vi "LoadFromLVSET.vi"(8 "Error In":errorcluster, 10 "No of Active\nModules":i32=1, 11 "File Path":path) -> (0 "Error Out":errorcluster, 3 "System Paramters For Each Module":T1[](array[typedef]) {"sync_freq_div" items=["1"=1, "2"=2, "4"=4]; "cfd_zc_level" min=-96 max=96 step=0.1 format="%#_3g"; "cfd_limit_low" min=-500 max=0 step=0.1 format="%#_3g"; "sync_zc_level" min=-96 max=96 step=0.1 format="%#_3g"; "sync_threshold" min=-500 max=-20 step=0.1 format="%#_3g"; "tac_limit_low" format="%.3g"; "tac_limit_high" min=0 max=100 step=0.1 format="%.3g"; "collect_time" min=1e-07 max=100000 step=0.001; "tac_offset" min=0 max=100 step=0.1 format="%.4g"; "tac_gain" min=1 max=15 step=1; "tac_range" format="%^#_6g"})   [LabVIEW 2017]
doc: "This convenience VI loads the user setting parameter such as TAC range, Sync Threshold and CFD Limit Low from a given LVSET file.\nIs no file specified the default file will be used, located at: \"C:\\BHdata\\SPCM\\SPCDefaultVal.lvset\"\n\ninfo@becker-hickl.com"
uses:
  Example_Controls/UserInput.ctl
panel:
  # "TAC / Time Range"
  # "CFD"
  # "(start)"
  # "SYNC"
  # "(stop)"
  # "range"
  # "gain"
  # "threshold(LL)"
  # "offset"
  # "limit high"
  # "limit low"
  # "zero cross(ZC)"
  # "Collection Time"
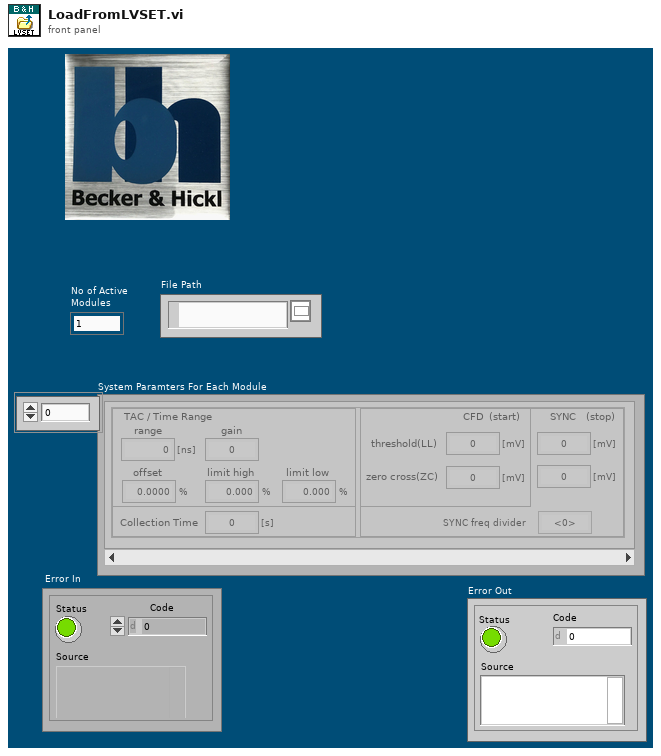
[diagram p1: front panel]
types:
  T1 = typedef "UserInput.ctl" = cluster{"tac_range":sgl, "tac_gain":i16, "tac_offset":sgl, "tac_limit_high":sgl, "tac_limit_low":sgl, "collect_time":sgl, "sync_threshold":sgl, "sync_zc_level":sgl, "sync_freq_div":i16, "cfd_limit_low":sgl, "cfd_zc_level":sgl}
  T2 = enum16{"open", "replace", "create", "open or create", "replace or create", "replace or create with confirmation"}
  T3 = enum16{"big-endian, network order", "native, host order", "little-endian"}
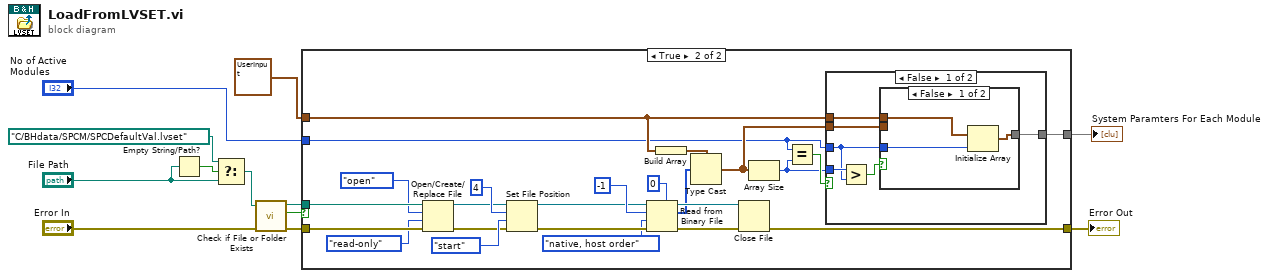
[diagram p0: block diagram]
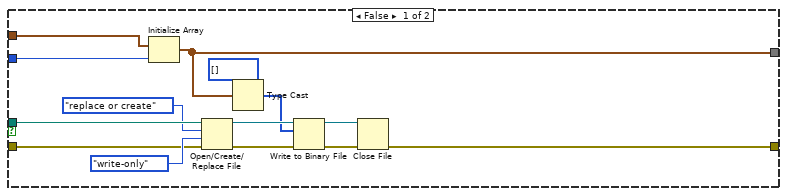
[diagram p2: hidden frame]
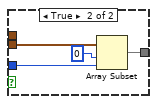
[diagram p3: hidden frame]
diagram:
  n1 = Empty String/Path?(string/path="File Path") -> (empty?=w6:bool)
  n2 = Select(t=path "C:/BHdata/SPCM/SPCDefaultVal.lvset", s=w6, f="File Path") -> (s? t:f=w4:path)
  n3 = call <vilib>:"Check if File or Folder Exists.vi"("error in (no error)"="Error In", "path"=w4) -> ("error out"=w2:errorcluster, "file or folder exists?"=w11:bool, "dup path"=w12:path)  [unwired: 7 in]
  n4 = case shown="True" w11 {
    tunnel: w12 -> [w24 w50]
    tunnel: w2 -> [w21 w49]
    tunnel: [w13 w33] -> w10
    tunnel: [w16 w32] -> w8
    tunnel: T1 {"tac_range"=50.0, "tac_gain"=1, "tac_offset"=0.0, "tac_limit_high"=10.0, "tac_limit_low"=80.0, "collect_time"=0.01, "sync_threshold"=-20.0, "sync_zc_level"=5.0, "sync_freq_div"=1, "cfd_limit_low"=1.0, "cfd_zc_level"=0.0} ("User Input") -> [w25 w29]
    tunnel: "No of Active\nModules" -> [w26 w28]
    frame False {
      n5 = Initialize Array(w25, w26) -> (w13:T1[])
      n6 = Open/Create/Replace File(file path (use dialog)=w24, error in=w21, operation (0:open)=T2."replace or create", access (0:read/write)=enum16{"read/write", "read-only", "write-only"}."write-only") -> (refnum out=w20:refnum<file>, error out=w19:errorcluster)  [unwired: 2 in, 1 out]
      n7 = Type Cast(type=u8[] [], x=w13) -> (*(type *) &x=w14:u8[])
      n8 = Write to Binary File(file (use dialog)=w20, data=w14, error in=w19) -> (refnum out=w18:refnum<file>, error out=w17:errorcluster)  [unwired: 3 in, 1 out]
      n9 = Close File(refnum=w18, error in=w17) -> (error out=w16:errorcluster)  [unwired: 1 out]
    }
    frame True {
      n10 = Open/Create/Replace File(file path (use dialog)=w50, error in=w49, operation (0:open)=T2."open", access (0:read/write)=enum16{"read/write", "read-only", "write-only"}."read-only") -> (refnum out=w46:refnum<file>, error out=w45:errorcluster)  [unwired: 2 in, 1 out]
      n11 = Set File Position(offset (in bytes) (0)=i64 4, refnum=w46, from (0:start)=enum16{"start", "end", "current"}."start", error in=w45) -> (refnum out=w41:refnum<file>, error out=w42:errorcluster)
      n12 = Read from Binary File(5:u8 0 ("Numeric"), 8:w42, 9:T3."native, host order" ("byte order (0:big-endian, network order)"), 10:-1 ("count (1)"), 11:w41) -> (0:w39:errorcluster, 2:w37:u8[], 3:w40:refnum<file>)  [unwired: 1 in, 1 out]
      n13 = Build Array(w29) -> (w27:T1[])
      n14 = Type Cast(type=w27, x=w37) -> (*(type *) &x=w34:T1[])
      n15 = Close File(refnum=w40, error in=w39) -> (error out=w32:errorcluster)  [unwired: 1 out]
      n16 = Array Size(array=w34) -> (size(s)=w35:i32)
      n17 = Equal?(x=w28, y=w35) -> (x = y?=w36:bool)
      n18 = case shown="False" w36 {
        tunnel: w35 -> [w56 _]
        tunnel: w28 -> [w53 _]
        tunnel: w34 -> [w54 w64]
        tunnel: [w52 w64] -> w33
        tunnel: w29 -> [w51 _]
        frame False {
          n19 = Greater?(x=w56, y=w53) -> (0:w55:bool)
          n20 = case shown="False" w55 {
            tunnel: w54 -> [_ w63]
            tunnel: w53 -> [w59 w62]
            tunnel: [w58 w60] -> w52
            tunnel: w51 -> [w57 _]
            frame False {
              n21 = Initialize Array(w57, w59) -> (w58:T1[])
            }
            frame True {
              n22 = Array Subset(array=w63, index=0, length=w62) -> (w60:T1[])
            }
          }
        }
        frame True {
        }
      }
    }
  }
  "System Paramters For Each Module" <- w10
  "Error Out" <- w8
